vi "RedisTabNameIndex.vi"(6 "RedisTabExecute":refnum<vi>, 8 "OP":T1(ring)=enum."Get", 9 "Enable?":bool=TRUE, 10 "Script":string[][](array[string]), 11 "RedisTabName":string) -> (0 "RedisTableConditionS":string[](array[string]), 1 "Enable?S":bool[](array[boolean]), 2 "Scripts":cluster{"Script":string[][]}[](array[cluster]), 3 "RedisTabNameS":string[](array[string]), 4 "RedisTabExecuteS":refnum<vi>[](array[refnum]))   [LabVIEW 2020]
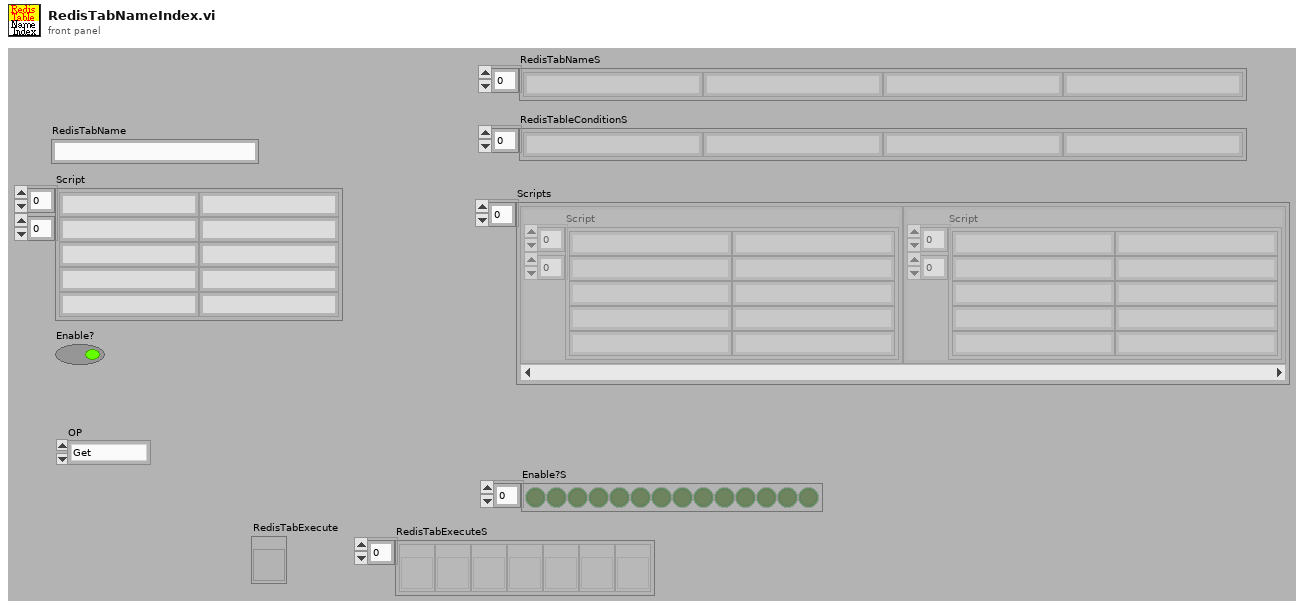
[diagram p1: front panel]
types:
  T1 = enum16{"Init", "Add", "Enable", "Disable", "Get", "UpdateVI"}
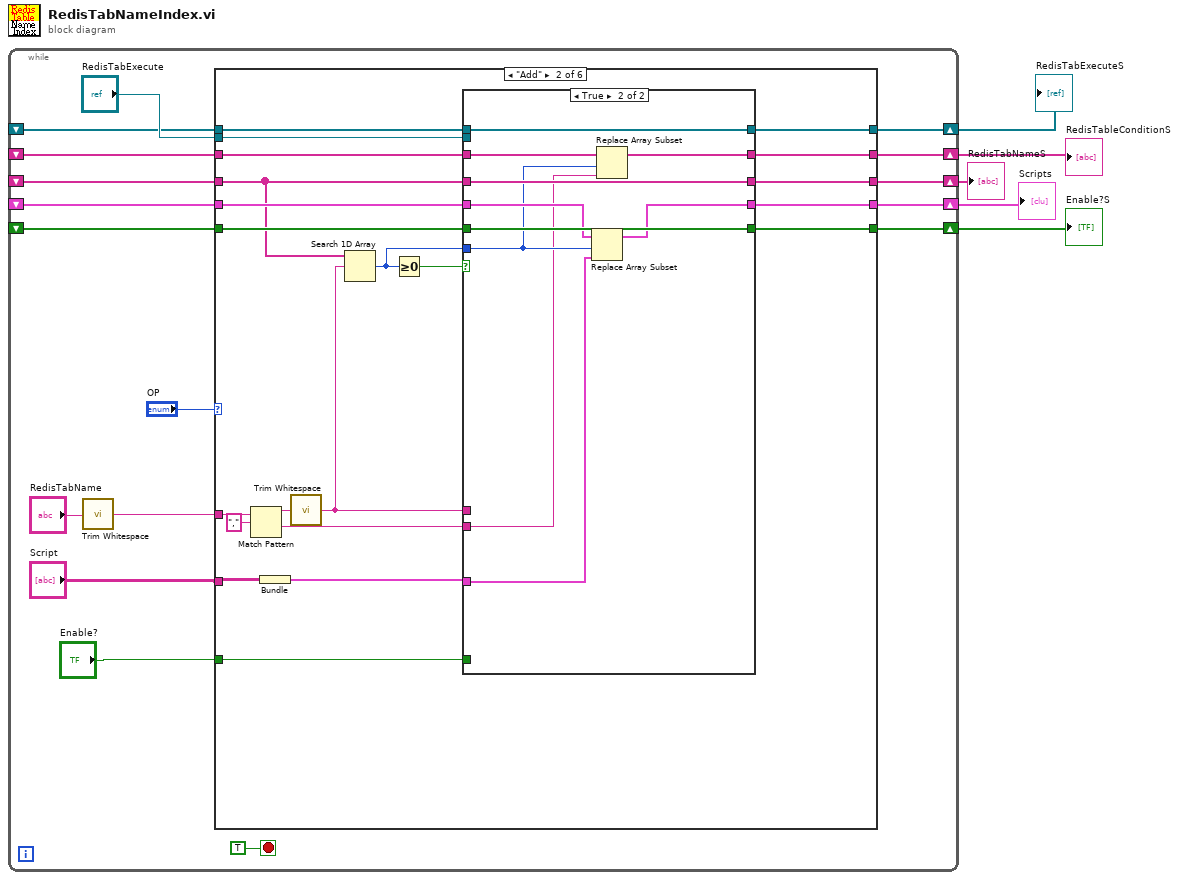
[diagram p0: block diagram]
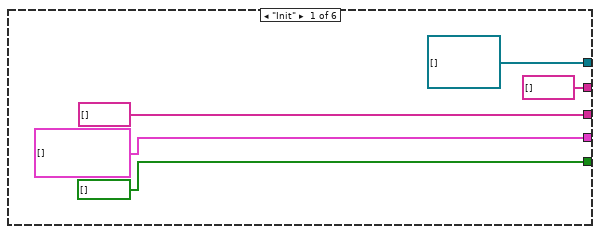
[diagram p2: hidden frame]
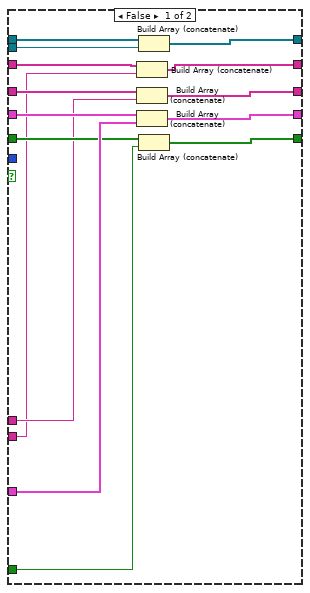
[diagram p3: hidden frame]
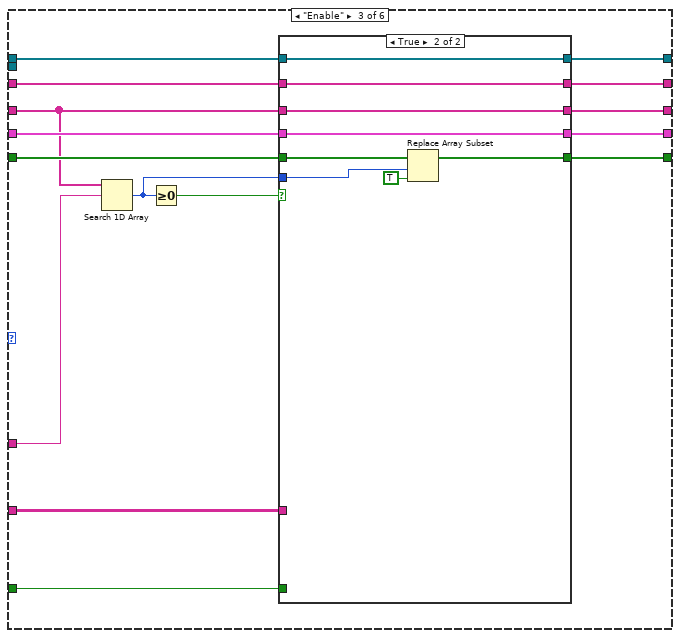
[diagram p4: hidden frame]
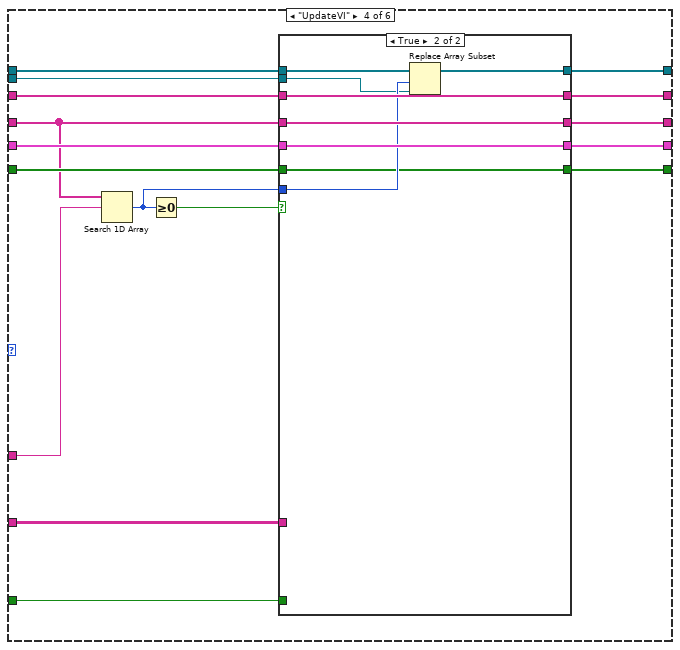
[diagram p6: hidden frame]
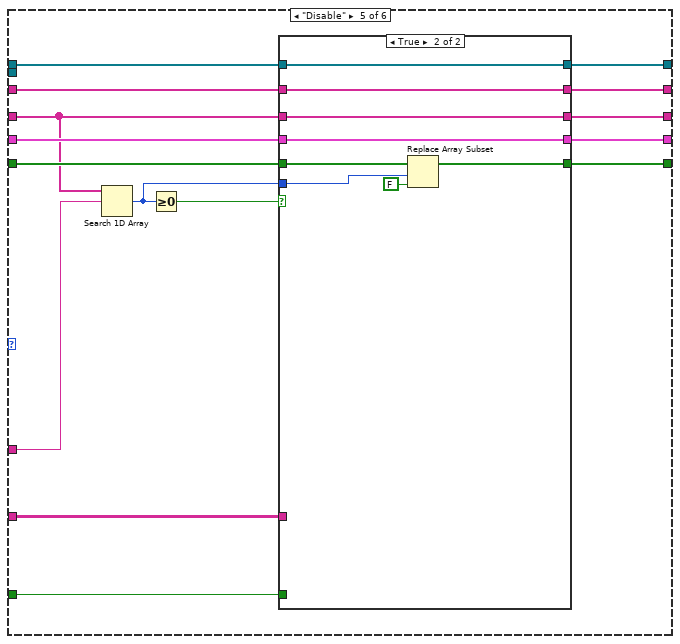
[diagram p8: hidden frame]
diagram:
  n1 = while {
    shift-right: [w20] -> w4
    shift-left: _ -> [w19]
    shift-right: [w18] -> w3
    shift-left: _ -> [w17]
    shift-right: [w14] -> w5
    shift-left: _ -> [w13]
    shift-right: [w10] -> w2
    shift-left: _ -> [w9]
    shift-right: [w8] -> w1
    shift-left: _ -> [w6]
    stop <- TRUE stop-if-true
    n2 = call <vilib>:"Trim Whitespace.vi"("string"="RedisTabName") -> ("trimmed string"=w15:string)  [unwired: 1 in]
    n3 = case shown="\"Add\"" "OP" {
      tunnel: "Script" -> [_ w39 w88 w117 w145 _]
      tunnel: "Enable?" -> [_ w43 w82 w111 w139 _]
      tunnel: [cluster{"Script":string[][]}[] [] w47 w86 w115 w143 w162] -> w20
      tunnel: w19 -> [_ w48 w87 w116 w144 w162]
      tunnel: [bool[] [] w46 w85 w114 w142 w161] -> w18
      tunnel: w17 -> [_ w45 w84 w113 w141 w161]
      tunnel: w15 -> [_ w37 w80 w109 w137 _]
      tunnel: [string[] [] w44 w83 w112 w140 w163] -> w14
      tunnel: w13 -> [_ w42 w81 w110 w138 w163]
      tunnel: [string[] [] w34 w76 w105 w133 w160] -> w10
      tunnel: w9 -> [_ w33 w77 w106 w134 w160]
      tunnel: [refnum<vi>[] [] w30 w74 w103 w131 w159] -> w8
      tunnel: "RedisTabExecute" -> [_ w29 _ w102 _ _]
      tunnel: w6 -> [_ w28 w75 w104 w132 w159]
      frame "Init" {
      }
      frame "Add" {
        n4 = Match Pattern(string=w37, regular expression=",") -> (before substring=w32:string, after substring=w35:string)  [unwired: 1 in, 2 out]
        n5 = Bundle("Script"=w39) -> (w38:cluster{"Script":string[][]})  [unwired: 1 in]
        n6 = call <vilib>:"Trim Whitespace.vi"("string"=w32) -> ("trimmed string"=w31:string)  [unwired: 1 in]
        n7 = Search 1D Array(1D array=w42, element=w31) -> (index of element=w40:i32)  [unwired: 1 in]
        n8 = Greater Or Equal To 0?(x=w40) -> (x >= 0?=w41:bool)
        n9 = case shown="True" w41 {
          tunnel: w38 -> [w63 w70]
          tunnel: w48 -> [w62 w71]
          tunnel: [w61 w69] -> w47
          tunnel: [w60 w72] -> w46
          tunnel: w45 -> [w59 w72]
          tunnel: [w58 w73] -> w44
          tunnel: w42 -> [w57 w73]
          tunnel: w43 -> [w56 _]
          tunnel: w40 -> [_ w67]
          tunnel: w31 -> [w55 _]
          tunnel: w35 -> [w54 w65]
          tunnel: [w53 w66] -> w34
          tunnel: w33 -> [w52 w68]
          tunnel: [w51 w64] -> w30
          tunnel: w29 -> [w50 _]
          tunnel: w28 -> [w49 w64]
          frame False {
            n10 = Build Array (concatenate)(w52, w54) -> (w53:string[])
            n11 = Build Array (concatenate)(w57, w55) -> (w58:string[])
            n12 = Build Array (concatenate)(w62, w63) -> (w61:cluster{"Script":string[][]}[])
            n13 = Build Array (concatenate)(w49, w50) -> (w51:refnum<vi>[])
            n14 = Build Array (concatenate)(w59, w56) -> (w60:bool[])
          }
          frame True {
            n15 = Replace Array Subset(array=w71, new element=w70, index=w67) -> (w69:cluster{"Script":string[][]}[])
            n16 = Replace Array Subset(array=w68, new element=w65, index=w67) -> (w66:string[])
          }
        }
      }
      frame "Enable" {
        n17 = Search 1D Array(1D array=w81, element=w80) -> (index of element=w78:i32)  [unwired: 1 in]
        n18 = Greater Or Equal To 0?(x=w78) -> (x >= 0?=w79:bool)
        n19 = case shown="True" w79 {
          tunnel: w88 -> [_ _]
          tunnel: w87 -> [w92 w99]
          tunnel: [w92 w99] -> w86
          tunnel: [w91 w97] -> w85
          tunnel: w84 -> [w91 w98]
          tunnel: [w93 w101] -> w83
          tunnel: w81 -> [w93 w101]
          tunnel: w82 -> [_ _]
          tunnel: w78 -> [_ w100]
          tunnel: w77 -> [w90 w95]
          tunnel: [w90 w95] -> w76
          tunnel: w75 -> [w89 w94]
          tunnel: [w89 w94] -> w74
          frame False {
          }
          frame True {
            n20 = Replace Array Subset(array=w98, new element=TRUE ("new element/subarray"), index=w100) -> (w97:bool[])
          }
        }
      }
      frame "UpdateVI" {
        n21 = Search 1D Array(1D array=w110, element=w109) -> (index of element=w107:i32)  [unwired: 1 in]
        n22 = Greater Or Equal To 0?(x=w107) -> (x >= 0?=w108:bool)
        n23 = case shown="True" w108 {
          tunnel: w117 -> [_ _]
          tunnel: w116 -> [w121 w129]
          tunnel: [w121 w129] -> w115
          tunnel: [w120 w123] -> w114
          tunnel: w113 -> [w120 w123]
          tunnel: [w122 w130] -> w112
          tunnel: w110 -> [w122 w130]
          tunnel: w111 -> [_ _]
          tunnel: w107 -> [_ w125]
          tunnel: w106 -> [w119 w128]
          tunnel: [w119 w128] -> w105
          tunnel: w104 -> [w118 w127]
          tunnel: [w118 w126] -> w103
          tunnel: w102 -> [_ w124]
          frame False {
          }
          frame True {
            n24 = Replace Array Subset(array=w127, new element=w124, index=w125) -> (w126:refnum<vi>[])
          }
        }
      }
      frame "Disable" {
        n25 = Search 1D Array(1D array=w138, element=w137) -> (index of element=w135:i32)  [unwired: 1 in]
        n26 = Greater Or Equal To 0?(x=w135) -> (x >= 0?=w136:bool)
        n27 = case shown="True" w136 {
          tunnel: w145 -> [_ _]
          tunnel: w144 -> [w149 w156]
          tunnel: [w149 w156] -> w143
          tunnel: [w148 w154] -> w142
          tunnel: w141 -> [w148 w155]
          tunnel: [w150 w158] -> w140
          tunnel: w138 -> [w150 w158]
          tunnel: w139 -> [_ _]
          tunnel: w135 -> [_ w157]
          tunnel: w134 -> [w147 w152]
          tunnel: [w147 w152] -> w133
          tunnel: w132 -> [w146 w151]
          tunnel: [w146 w151] -> w131
          frame False {
          }
          frame True {
            n28 = Replace Array Subset(array=w155, new element=FALSE ("new element/subarray"), index=w157) -> (w154:bool[])
          }
        }
      }
      frame "Get" {
      }
    }
  }
  "RedisTabNameS" <- w5
  "Scripts" <- w4
  "Enable?S" <- w3
  "RedisTableConditionS" <- w2
  "RedisTabExecuteS" <- w1
